vi "Create FC name.vi"(0 "reference in":refnum<class "metadata.lvclass">, 1 "Vel_app (nm/s)":dbl=0.1 min=3.0 max=5000000.0 step=1.0 format="%#.7f", 2 "Vel_ret (nm/s)":dbl=3.0 min=3.0 max=5000000.0 step=1.0 format="%#.7f", 5 "error in (no error)":errorcluster, 9 "# of scans":u32) -> (14 "reference out":refnum<class "metadata.lvclass">, 15 "Fcurve Name":string, 17 "current time":timestamp, 19 "error out":errorcluster)   [LabVIEW 2019, in "metadata.lvclass"]
uses:
  metadata.lvclass
  Write time and date string --constant.ctl
panel:
  out "result string":string
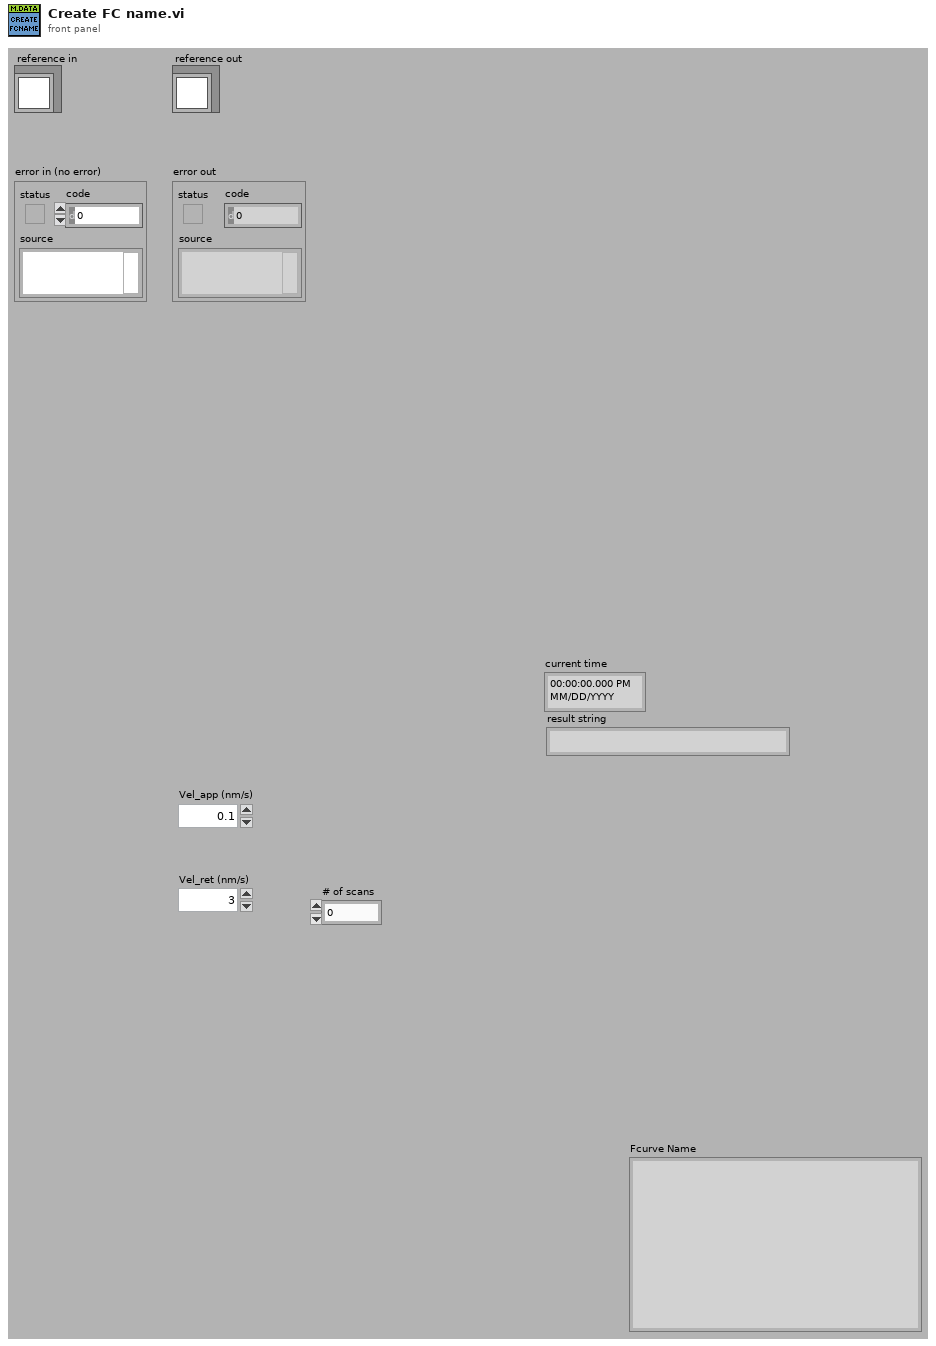
[diagram p1: front panel]
types:
  T1 = typedef "metadata.lvclass/Write time and date string --constant.ctl" = string
  T2 = typedef "metadata.lvclass/ObjectAttributesRef.ctl" = refnum<data-value>
  T3 = typedef "metadata.lvclass/ObjectAttributes.ctl" = cluster{"MyAttribute":dbl, "System Control":T4, "file info":T5, "Sample info":T6, "Cantilever info":T7, "XYZ piezos":T8, "Mapping":T9, "Fcurve segment":T10[], "Fast fpga segment":T12, "Chirp":T13, "precision (6)":i16, "width (-)":i16, "Metadata":T14, "config filepath":path, "Section names []":string[], "Property names []":string[], "nb elements":u16}
  T4 = typedef "metadata.lvclass/System control parameters.ctl" = cluster{"FPGA SW version":string, "TDMS file version":string, "Instrument":string, "Instrument model":string, "Instrument scanner":string, "Instrument clockrate (Mhz)":string, "Instrument tick time (us)":string}
  T5 = typedef "metadata.lvclass/File info parameters.ctl" = cluster{"Time Stamp":timestamp, "Filename":string, "Filepath":path, "User":string, "Experiment_name":string, "Curve_id":string, "number_segments":u8, "number_consecutive_scans":u32}
  T6 = typedef "metadata.lvclass/Sample info parameters.ctl" = cluster{"Sample name":string, "Sample species":string}
  T7 = typedef "metadata.lvclass/Cantilever info parameters.ctl" = cluster{"spring constant calib method":string, "invOLS calib method":string, "thermal calib deflection channel":string, "model":string, "shape":string, "tip geometry":string, "Laser sum (V)":dbl, "Laser power (mA)":dbl, "invOLS_(nm/V)":dbl, "spring constant nominal (N/m)":dbl, "spring constant calib (N/m)":dbl, "resosnance frequency air calib (Hz)":dbl, "resosnance frequency calib (Hz)":dbl, "quality factor":dbl, "Acoefficident_GCI_(nN.s^1.3/m)":dbl, "half angle (deg)":dbl, "tip radius (m)":dbl, "tip height (m)":dbl, "system mount angle (deg)":dbl}
  T8 = typedef "metadata.lvclass/XYZ piezos parameters.ctl" = cluster{"X stage piezo sensitivity (nm/V)":dbl, "X stage piezo gain":dbl, "X velocity (V/tick)":dbl, "X closed loop":bool, "Y stage piezo sensitivity (nm/V)":dbl, "Y stage piezo gain":dbl, "Y velocity (V/tick)":dbl, "Y closed loop":bool, "Z stage piezo sensitivity (nm/V)":dbl, "Z stage piezo gain":dbl, "Z closed loop":bool, "X position (V)":dbl, "Y position (V)":dbl}
  T9 = typedef "metadata.lvclass/Mapping parameters.ctl" = cluster{"Mapping":bool, "index":u16, "position row":u16, "position column":u16, "next position row":i16, "next position column":i16, "X initial position (V)":dbl, "Y initial position (V)":dbl, "X step size (V)":dbl, "Y step size (V)":dbl}
  T10 = typedef "metadata.lvclass/Fcurve segment.ctl" = cluster{"type":T11, "fast_fpga_trigger":bool, "nb":u8, "duration (ticks)":i64, "nb points":i32, "sampling rate (S/s)":u32, "Zpiezo control out":string, "initial deflection (V)":dbl, "relative setpoint":bool, "setpoint on":bool, "setpoint (V)":dbl, "setpoint trigger channel":string, "velocity (V/tick)":dbl, "Z position setpoint trigger (V)":dbl, "Z retract length (V)":dbl, "dec factor":u32}
  T11 = typedef "metadata.lvclass/Segment type--combobox.ctl" = string
  T12 = typedef "metadata.lvclass/fast fpga segment parameters.ctl" = cluster{"Fast start time trigger":timestamp, "nb_points":u32, "sampling_rate_(S/s)":u32, "duration_(ticks)":u32}
  T13 = typedef "metadata.lvclass/Chirp added parameters.ctl" = cluster{"f start (Hz)":dbl, "f end (Hz)":dbl, "Sweep type":string}
  T14 = typedef "metadata.lvclass/Metadata output --cluster.ctl" = cluster{"Property Names":string[], "Property Values":variant[]}
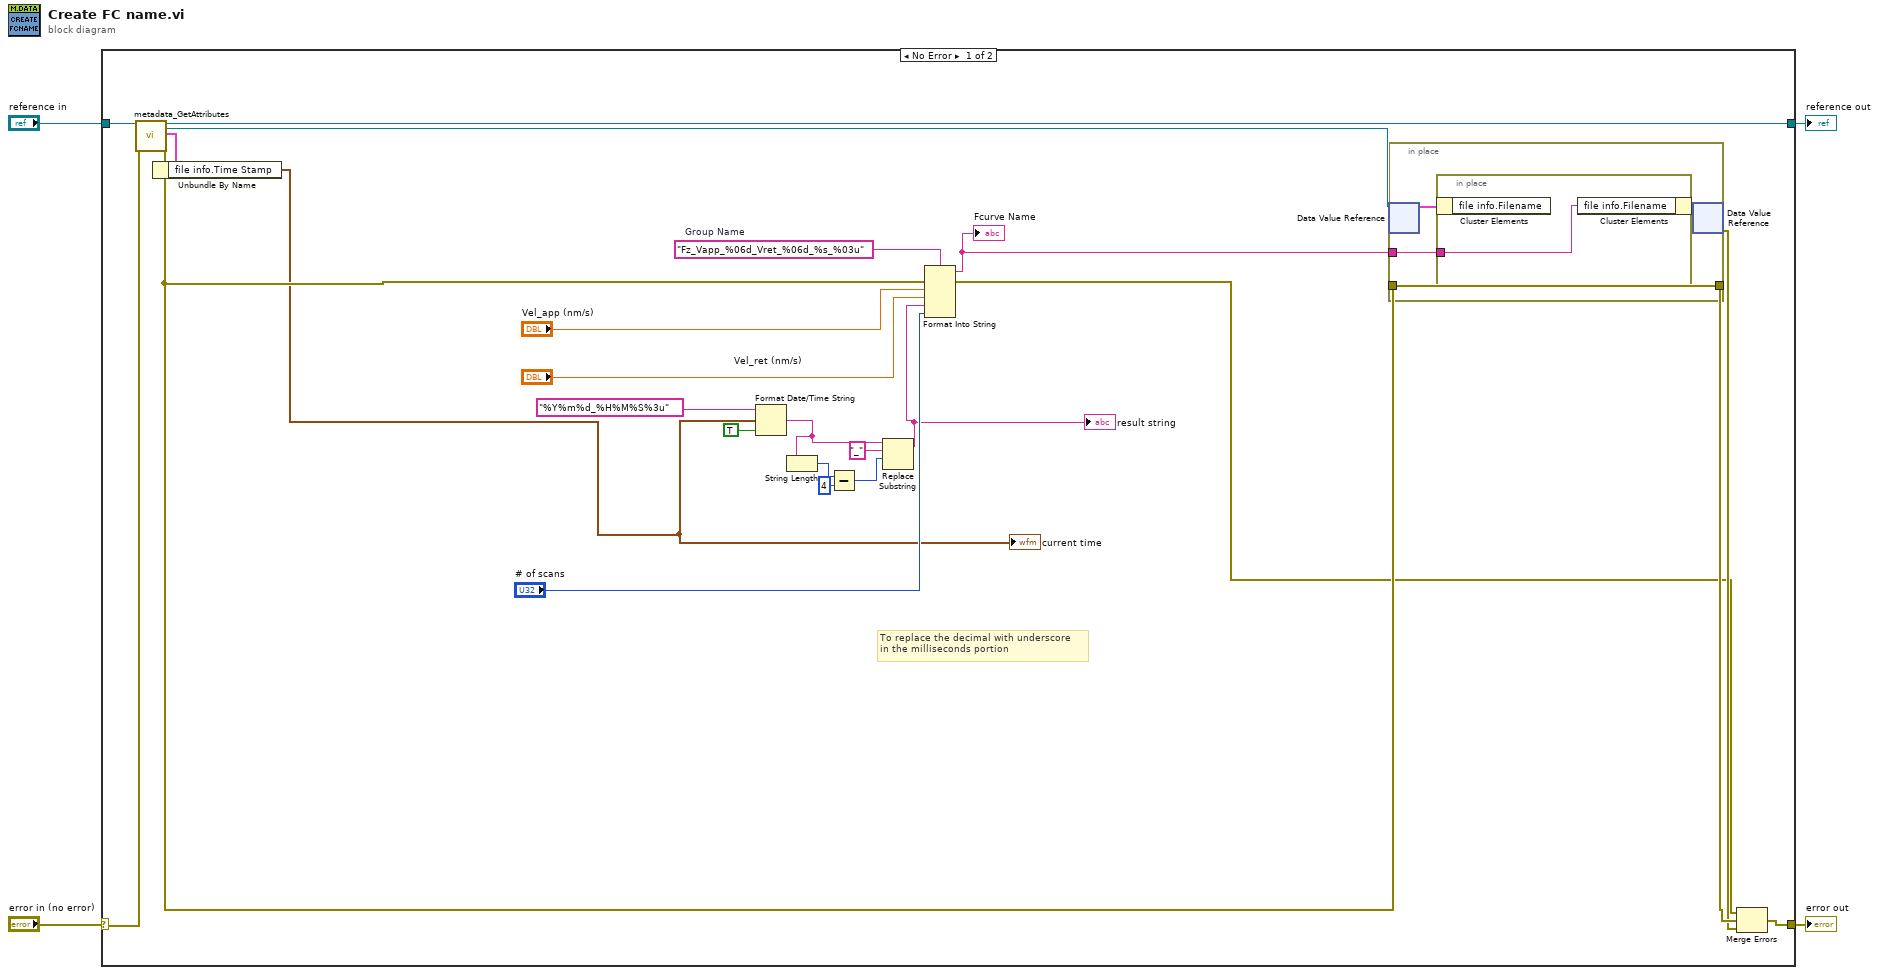
[diagram p0: block diagram]
diagram:
  n1 = case shown="No Error" "error in (no error)" {
    selector: "error in (no error)" -> [w25 w35]
    tunnel: [w28 w35] -> w3
    tunnel: [w26 w34] -> w1
    tunnel: "reference in" -> [w27 w34]
    frame No Error {
      w20 = "Fz_Vapp_%06d_Vret_%06d_%s_%03u"  # Group Name
      # "To replace the decimal with underscore\nin the milliseconds portion"
      n2 = call "metadata_GetAttributes.vi"("reference in"=w27, "error in (no error)"=w25) -> ("reference out"=w26:refnum<class "metadata.lvclass">, "attributes ref"=w21:T2, "attributes"=w24:T3, "error out"=w9:errorcluster)  [unwired: 14 in]
      n3 = Unbundle By Name(w24) -> ("file info.Time Stamp"=w6:timestamp)
      "current time" <- w6
      n4 = Format Date/Time String(time format string (%c)=T1 "%Y%m%d_%H%M%S%3u", seconds (now)=w6, UTC format=TRUE) -> (date/time string=w14:string)
      n5 = String Length(string=w14) -> (length=w13:i32)
      n6 = Subtract(x=w13, y=4) -> (x-y=w11:i32)
      n7 = Replace Substring(3:w11, 4:"_" ("substring (\"\")"), 5:w14) -> (1:w10:string)  [unwired: 1 in, 1 out]
      "result string" <- w10
      n8 = Format Into String(format string=w20, error in=w9, "Vel_app (nm/s)", "Vel_ret (nm/s)", w10, "# of scans") -> (resulting string=w5:string, error out=w8:errorcluster)  [unwired: 1 in]
      "Fcurve Name" <- w5
      n9 = in-place {
        in-place-border: w9 -> [w30]
        in-place-border: [w30] -> w23
        in-place-border: w5 -> [w29]
        n10 = in-place-dvr #1(w21) -> (w31:T3)  [unwired: 1 out]
        n11 = in-place {
          in-place-border: w29 -> [w33]
          n12 = in-place-cluster #2(w31) -> ()  [unwired: 1 out]
          n13 = in-place-cluster #2("file info.Filename"=w33) -> (w32:T3)
        }
        n14 = in-place-dvr #1(w32) -> (w22:errorcluster)  [unwired: 1 out]
      }
      n15 = Merge Errors(w8, w23, w22) -> (w28:errorcluster)
    }
    frame Error {
    }
  }
  "error out" <- w3
  "reference out" <- w1
